vi "tan_45_to_45.vi"(1 "theta":i8) -> (0 "tan(theta)":fxp<+/-,16,1> format="%.16g")   [LabVIEW 2010]
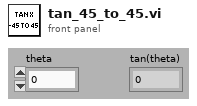
[diagram p1: front panel]
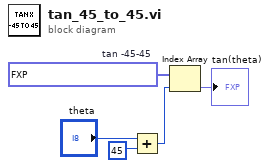
[diagram p0: block diagram]
diagram:
  w1 = fxp<+/-,16,1>[] [-1.0, -0.9656982421875, -0.932525634765625, -0.900390625, -0.869293212890625, -0.839111328125, -0.809783935546875, -0.781280517578125, -0.7535400390625, -0.726531982421875, -0.7001953125, -0.67449951171875, -0.6494140625, -0.6248779296875, -0.600860595703125, -0.577362060546875, -0.5543212890625, -0.531707763671875, -0.509521484375, -0.48773193359375, -0.46630859375, -0.445220947265625, -0.424468994140625, -0.404022216796875, -0.38385009765625, -0.363983154296875, -0.344329833984375, -0.324920654296875, -0.30572509765625, -0.2867431640625, -0.2679443359375, -0.24932861328125, -0.230865478515625, -0.212554931640625, -0.194366455078125, -0.17633056640625, -0.15838623046875, -0.140533447265625, -0.122772216796875, -0.1051025390625, -0.087493896484375, -0.069915771484375, -0.052398681640625, -0.034912109375, -0.0174560546875, 0.0, 0.0174560546875, 0.034912109375, 0.052398681640625, 0.069915771484375, 0.087493896484375, 0.1051025390625, 0.122772216796875, 0.140533447265625, 0.15838623046875, 0.17633056640625, 0.194366455078125, 0.212554931640625, 0.230865478515625, 0.24932861328125, 0.2679443359375, 0.2867431640625, 0.30572509765625, 0.324920654296875, 0.344329833984375, 0.363983154296875, 0.38385009765625, 0.404022216796875, 0.424468994140625, 0.445220947265625, 0.46630859375, 0.48773193359375, 0.509521484375, 0.531707763671875, 0.5543212890625, 0.577362060546875, 0.600860595703125, 0.6248779296875, 0.6494140625, 0.67449951171875, 0.7001953125, 0.726531982421875, 0.7535400390625, 0.781280517578125, 0.809783935546875, 0.839111328125, 0.869293212890625, 0.900390625, 0.932525634765625, 0.9656982421875, 0.0]  # tan -45-45
  n1 = Add(x="theta", y=u8 45) -> (x+y=w3:u8)
  n2 = Index Array(array=w1, index=w3) -> (element=→"tan(theta)":fxp<+/-,16,1>)
